vi "DAQ Get Analog Input.vi"(8 "error in (no error)":errorcluster, 10 "Samples":i32, 11 "Waveforms In":waveform(dbl)[](array[waveform])) -> (0 "error out":errorcluster, 3 "Waveforms Out":waveform(dbl)[](array[waveform]))   [LabVIEW 2017]
doc: "This VI acquires new data from PrecorAI task and add it to the end of array of waveforms.\n\nI didn't have to make a subVI for this, but it starts to get cluttered at DAQ Loop VI so I made one"
uses:
  <vilib>/DAQmx/read.llb/DAQmx Read (Analog 1D Wfm NChan NSamp).vi
  <vilib>/DAQmx/miscellaneous.llb/DAQmx Fill In Error Info.vi
  <vilib>/Waveform/WDTOps.llb/WDT Append Waveforms DBL.vi
  <vilib>/Waveform/WDTOps.llb/WDT Get Waveform Subset DBL.vi
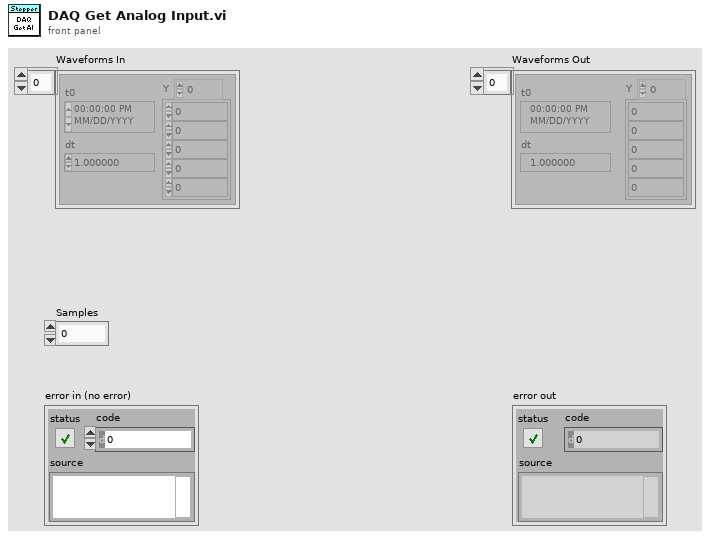
[diagram p1: front panel]
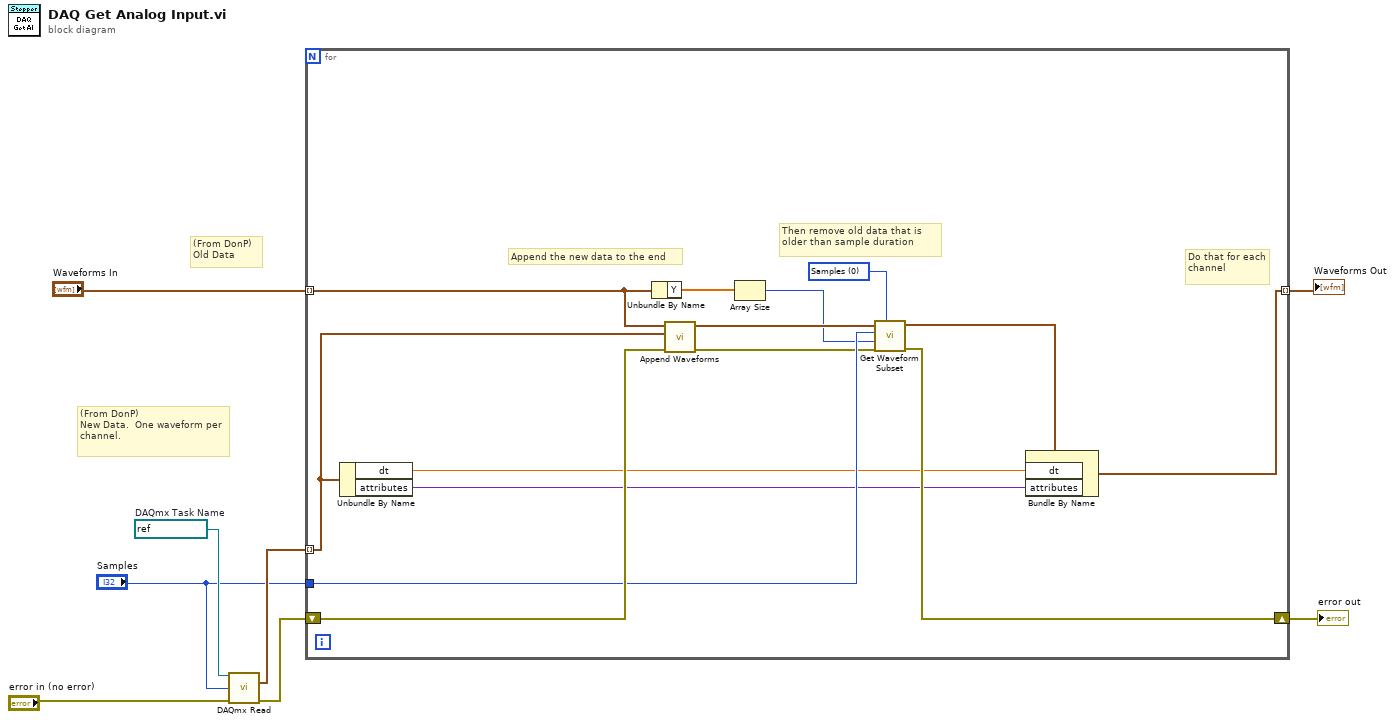
[diagram p0: block diagram]
diagram:
  w8 = refnum<k21> "PrecorAI"  # DAQmx Task Name
  # "(From DonP)\nNew Data.  One waveform per channel."
  # "(From DonP)\nOld Data"
  n1 = call-poly <vilib>:"DAQmx Read.vi"("task/channels in"=w8, "number of samples per channel"="Samples", "error in"="error in (no error)") -> ("data"=w7:waveform(dbl)[], "error out"=w6:errorcluster)  [unwired: 10 in, 1 out]
  n2 = for {
    tunnel: w7 -> [w16] mode=indexing
    tunnel: "Waveforms In" -> [w11] mode=indexing
    tunnel: [w12] -> w3 mode=indexing
    shift-right: [w17] -> w1
    shift-left: w6 -> [w22]
    tunnel: "Samples" -> [w20]
    w18 = u16 0 items=["Samples", "Relative Time"] ("start/duration format")
    # "Do that for each channel"
    # "Then remove old data that is older than sample duration"
    # "Append the new data to the end"
    n3 = Unbundle By Name(w16) -> ("dt"=w14:dbl, "attributes"=w13:variant)
    n4 = Unbundle By Name(w11) -> ("Y"=w10:dbl[])
    n5 = call-poly <vilib>:"Append Waveforms.vi"("error in (no error)"=w22, "waveform B"=w16, "waveform A"=w11) -> ("error out"=w19:errorcluster, "waveform out"=w21:waveform(dbl))  [unwired: 7 in]
    n6 = Array Size(array=w10) -> (size(s)=w9:i32)
    n7 = call-poly <vilib>:"Get Waveform Subset.vi"("start/duration format"=w18, "error in (no error)"=w19, "duration"=w9, "start samples/time"=w20, "waveform in"=w21) -> ("error out"=w17:errorcluster, "waveform out"=w15:waveform(dbl))  [unwired: 1 in, 2 out]
    n8 = Bundle By Name(cluster=w15, "dt"=w14, "attributes"=w13) -> (w12:waveform(dbl))
  }
  "Waveforms Out" <- w3
  "error out" <- w1
